vi "Vision.vi"() -> ()   [LabVIEW 2013]
uses:
  StateMachineStates 1.ctl
  <vilib>/DAQmx/read.llb/DAQmx Read (Counter DBL 1Chan 1Samp).vi
  <vilib>/DAQmx/create/channels.llb/DAQmx Create Channel (CI-Pulse Width).vi
  <vilib>/DAQmx/miscellaneous.llb/DAQmx Fill In Error Info.vi
panel:
  out "Triggered":bool
  in  "Use EEG trigger?":bool
  in  "Entrainment":bool=TRUE
  in  "Sound at \nstimulus end":bool
  in  "Manual \nvoltage (V)":dbl=2.6 format="%.2p"
  in  "Manual \nphoton #":i64=100
  out "L/R WP target":dbl
  out "List of axes":i32[](array[numeric])
  out "List of WP errors":bool[](array[boolean])
  out "WP error":bool
  out "appended array":dbl[][](array[numeric])
  out "Pump WP":dbl format="%.2f"
  in  "Trigger rate at \n52.6 degrees":dbl=2646.0 format="%.2p"
  in  "Target trial \nlength (ms)":dbl=500.0 format="%.2p"
  in  "Default pump \nWP angle":dbl=52.6
  in  "Pump WP":bool=TRUE
  out "Photon time (ms)":dbl format="%.2f"
  in  "Interval (ms)":u32
  out "Repetition":dbl
  in  "Repetitions":dbl=1.0
  out "WP time (ms)":u32
  out "VISA Handle out":refnum<visa-resource-name>="ASRL5::INSTR"
  out "Initializing":bool
  out "Trial mode":enum16{"Single Photons", "LED", "Mixed LED"}(ring)
  in  "Frequency of LED trials\nfor Mixed mode":dbl=30.0
  out "Bright trial\nrequested":bool
  out "Observer Ready":bool
  in  "Bright/mixed mode \nLED voltage (V)":dbl=2.6 min=-3.0 max=4.0 format="%.2f"
  in  "GPIB address":string="15"
  in  "Period (ms)":i64=20
  in  "Pulse \nlength (ms)":dbl=50.0
  out "L/R WP":dbl format="%.2f"
  in  "Manually \ninitialize":bool
  in  "COM for WPs":u8=3
  out "Blocked trial #":i32
  out "Photon #":i32
  out "LED Voltage":dbl
  in  "Blocking requirements":cluster{"Value":dbl, " Number":i32}[](array[cluster])
  in  "Manual":bool
  in  "Path":path=path "C:/Users/lab/Dropbox/Research/Data/Vision"
  out "Counts 2":u32
  out "Counts 1":u32
  in  "Delay for APDs (ms)":u32=25
  in  "Counter 2":tag="Dev1/ctr1"
  in  "Counter 1":tag="Dev1/ctr0"
  out "Trial #":i32
  in  "Mode":enum16{"Single Photons", "LED", "Mixed"}(ring)=enum."Mixed"
  in  "Audio":bool=TRUE
  in  "Self-paced":bool
  out "Stimulus":bool
  out "Location Set":bool
  out "Stimulus \nlocation":string
  out "Waiting":bool
  out "Observer Responded":bool
  out "Response \ntime (ms)":dbl
  out "Observer \nchoice":string
  out "Confidence":i32
  in  "stop":bool
  in  "Next Trial":bool
  in  "Create New File":bool
  out "Subject #":string
  # "Settings for Blocking\nand Mixed Mode"
  # "Instructions: Run VI. Enter blocking requirements, then press\nCreate New File. Initialize waveplates if necessary, and set\nhighlighted controls to desired values. Press Next Trial to begin."
  # "Researcher Interface"
  # "Trial Options"
  # "Counter Options"
  # "Trial Information"
  # "(1)"
  # "(3)"
  # "LED Options"
  # "Pump Settings"
  # "Troubleshooting"
  # "Waveplates"
  # "(2)"
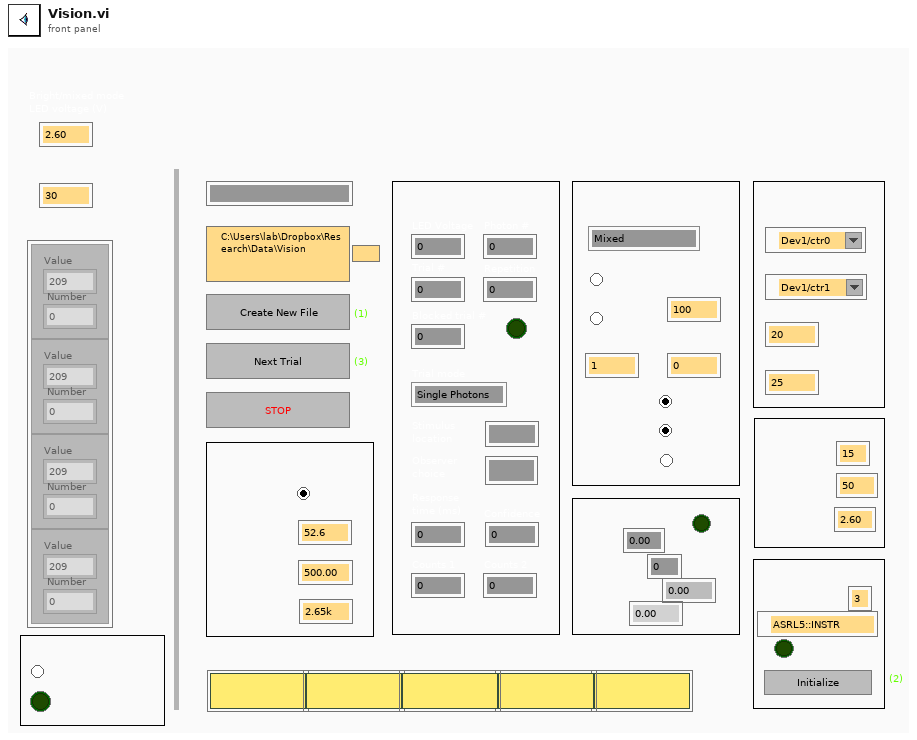
[diagram p1: front panel]
types:
  T1 = typedef "StateMachineStates 1.ctl" = enum16{"WaitResearcher", "Setup", "SetWP", "WaveplateError", "WaitObserverReady", "EEG", "Photons", "LED", "WaitObserverResponse", "CleanUp", "Stop"}
  T2 = enum16{"0", "1", "2", "3", "4", "5", "6", "7", "8", "9", "A", "B", "C", "D", "E", "F", "G", "H", "I", "J", "K", "L", "M", "N", "O", "P", "Q", "R", "S", "T", "U", "V", "W", "X", "Y", "Z", "F1", "F2", "F3", "F4", "F5", "F6", "F7", "F8", "F9", "F10", "F11", "F12", "F13", "F14", "F15", "ADD", "BACK", "BACKSLASH", "CAPITAL", "COMMA", "DECIMAL", "DELETE", "DIVIDE", "DOWN", "END", "EQUALS", "ESCAPE", "GRAVE (`)", "HOME", "INSERT", "LBRACKET", "LCONTROL", "LEFT", "L ALT", "LSHIFT", "LWIN", "MINUS", "MULTIPLY", "NEXT", "NUMLOCK", "NUMPAD_0", "NUMPAD_1", "NUMPAD_2", "NUMPAD_3", "NUMPAD_4", "NUMPAD_5", "NUMPAD_6", "NUMPAD_7", "NUMPAD_8", "NUMPAD_9", "PAUSE", "PERIOD", "PRIOR (PG UP)", "RBRACKET", "RCONTROL", "RETURN", "RIGHT", "R ALT", "RSHIFT", "RWIN", "SCROLL", "SEMICOLON", "SLASH", "SPACE", "SUBTRACT", "TAB", "UP", "ENTER (num pad)", "' (quote)"}
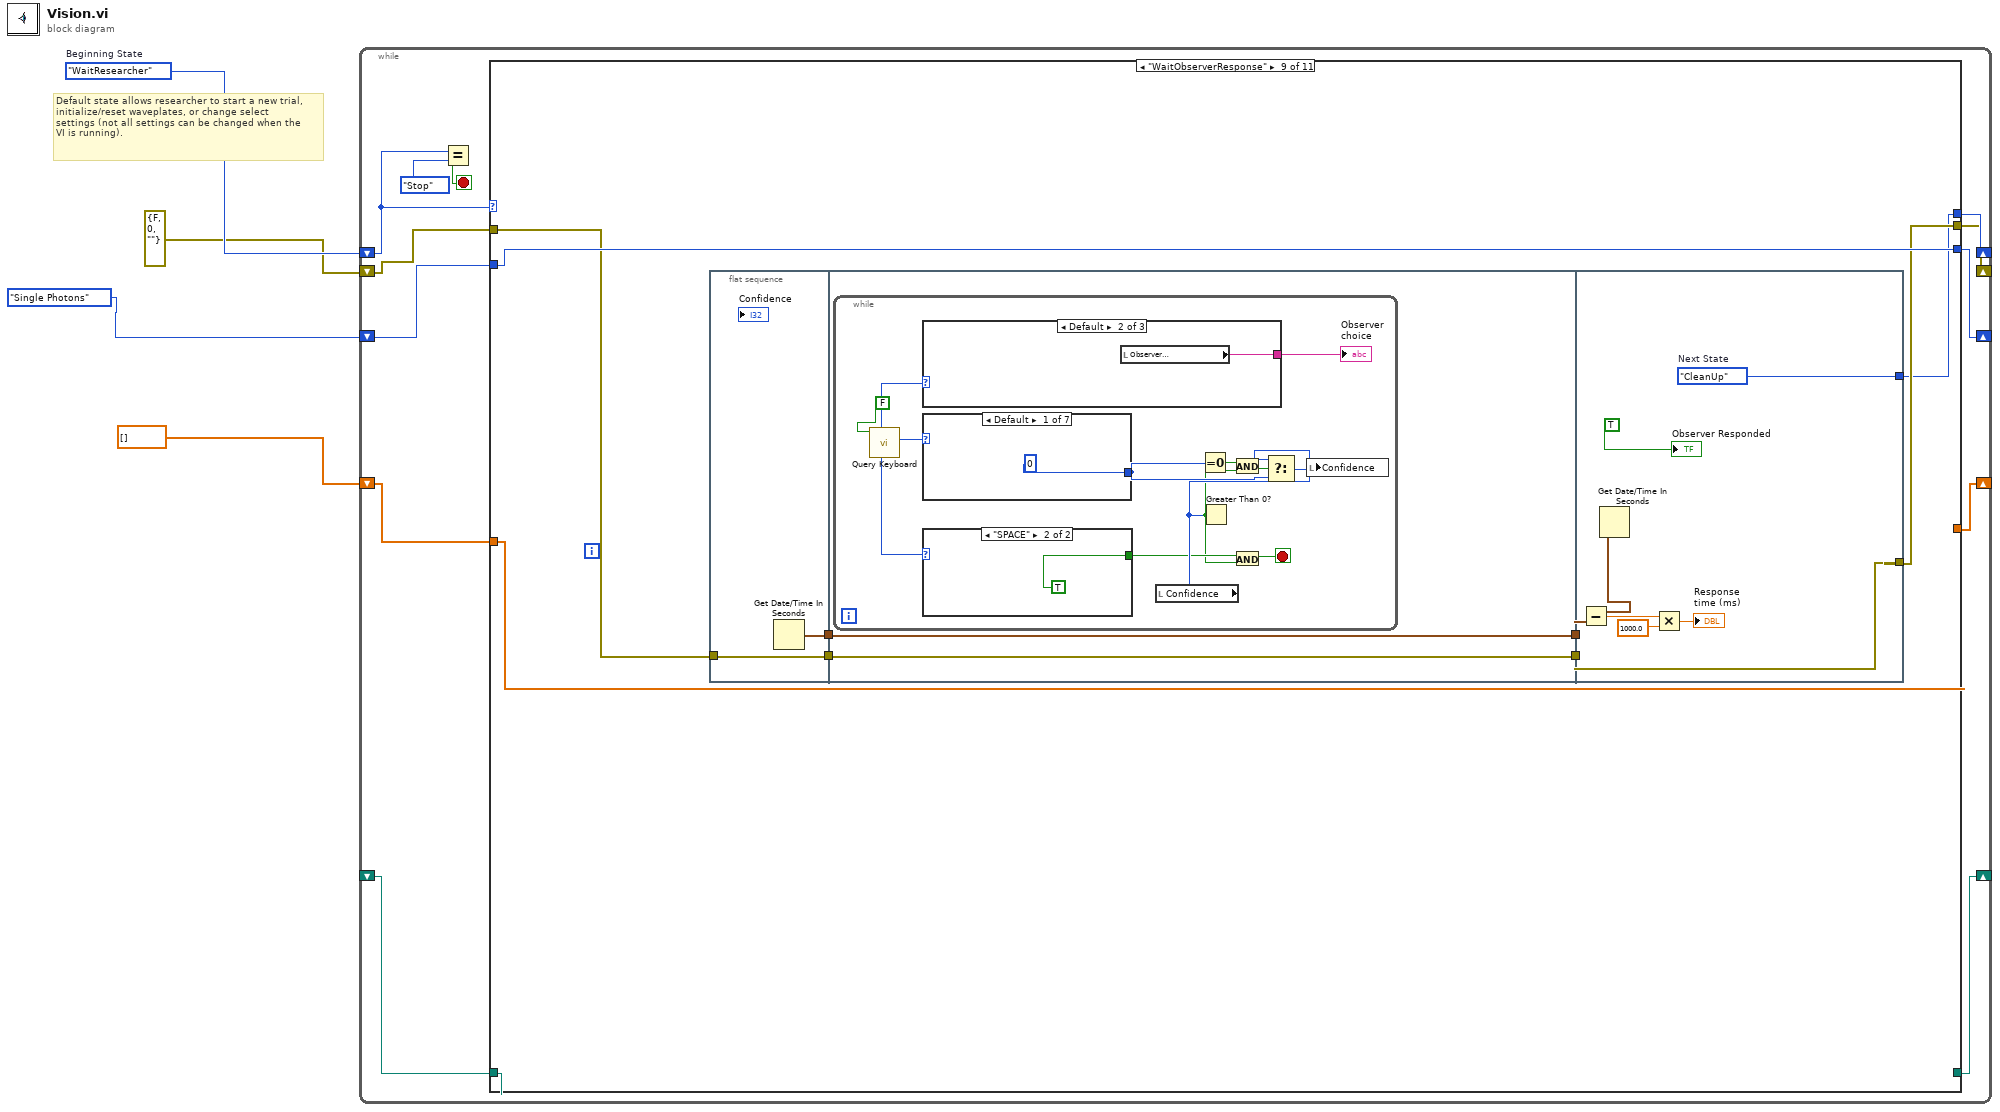
[diagram p0: block diagram]
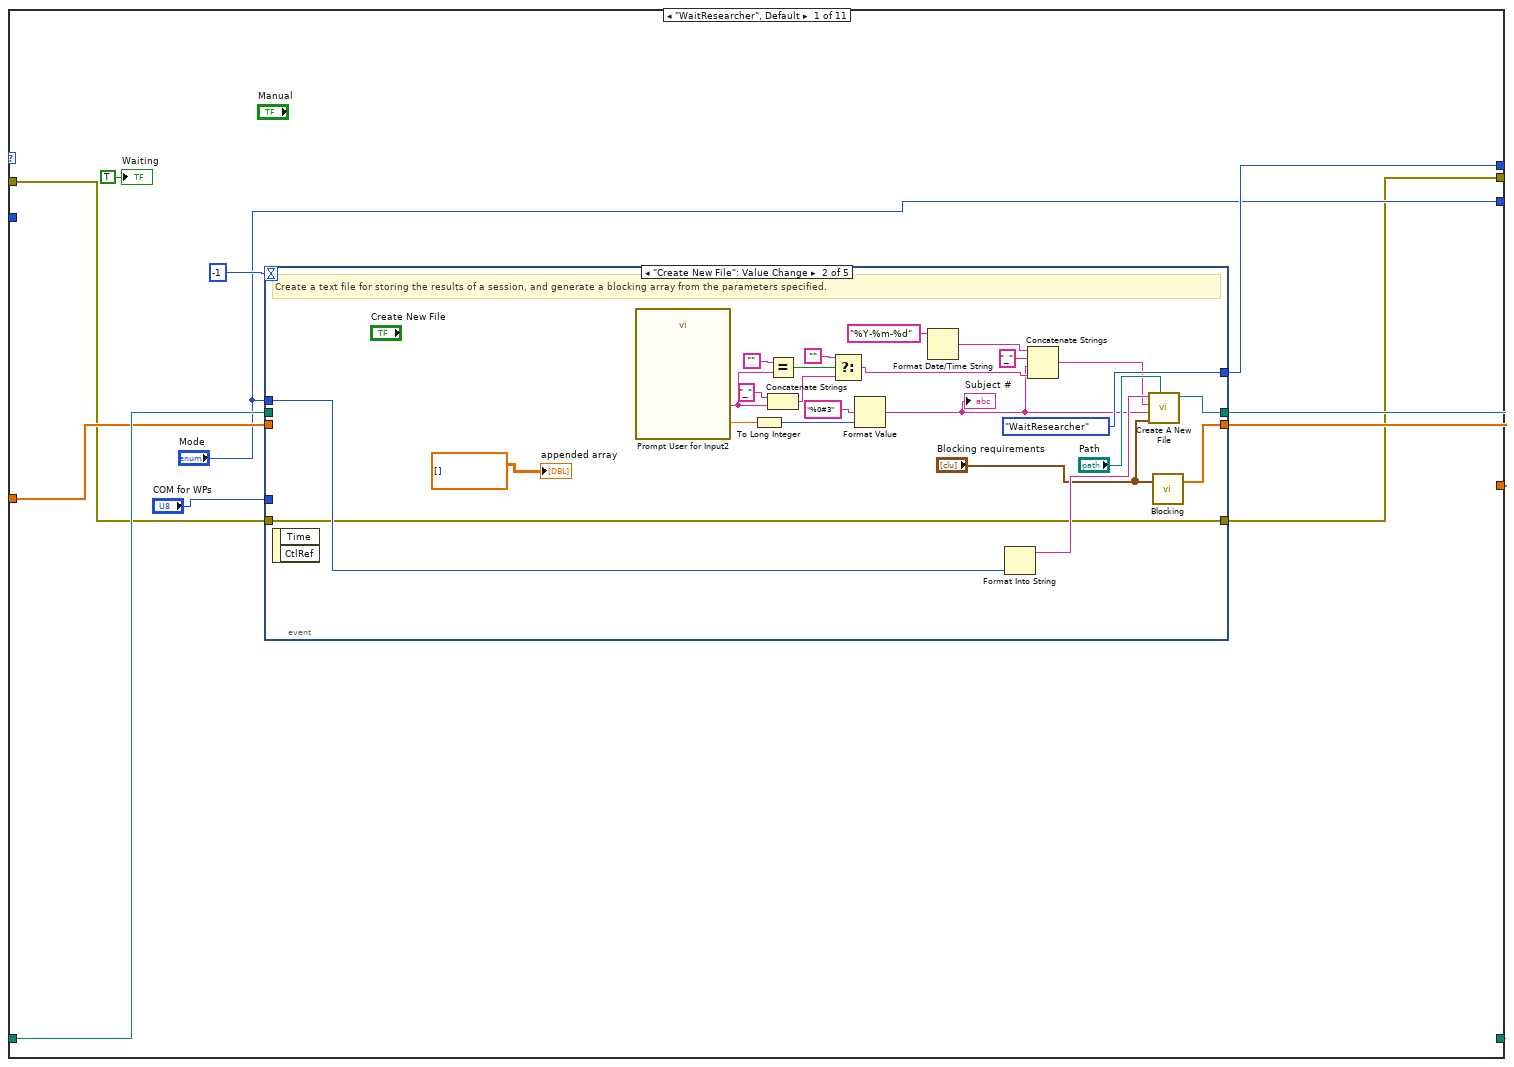
[diagram p2: hidden frame]
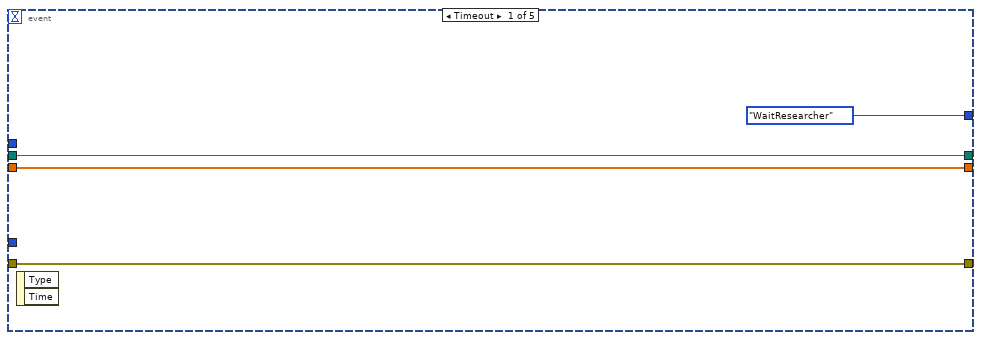
[diagram p3: hidden frame]
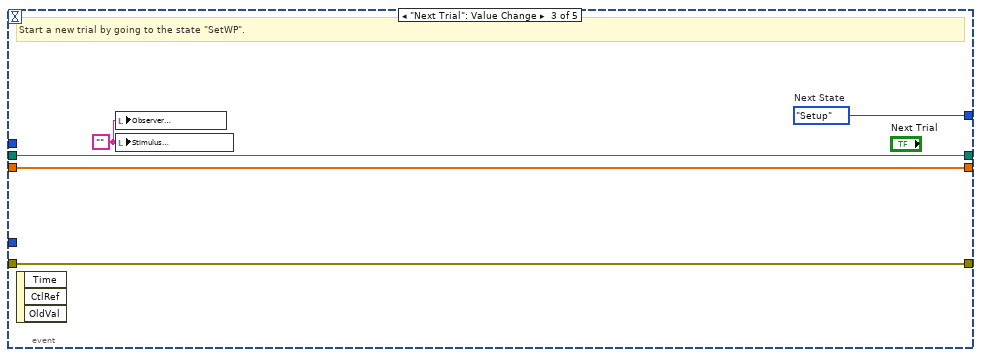
[diagram p4: hidden frame]
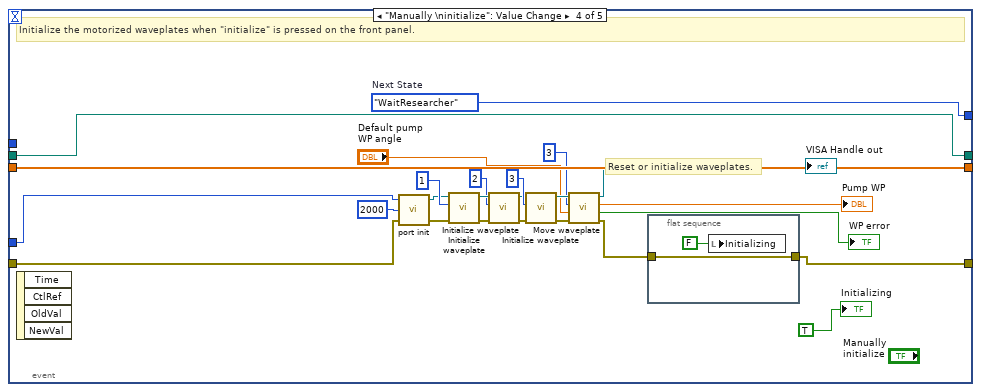
[diagram p5: hidden frame]
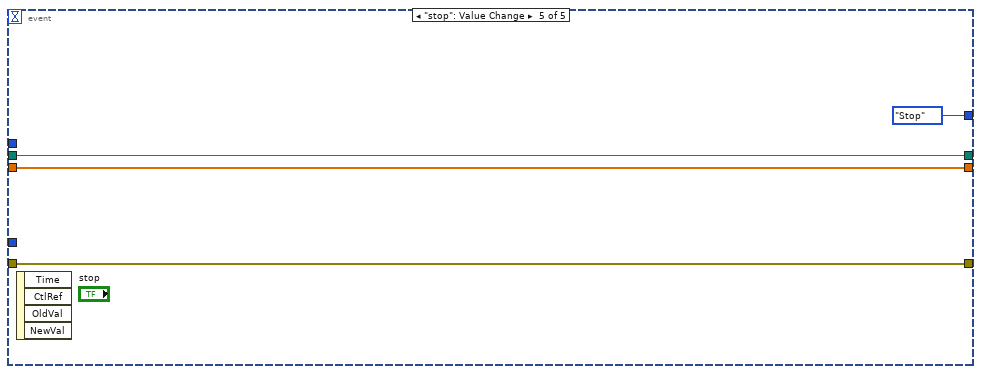
[diagram p6: hidden frame]
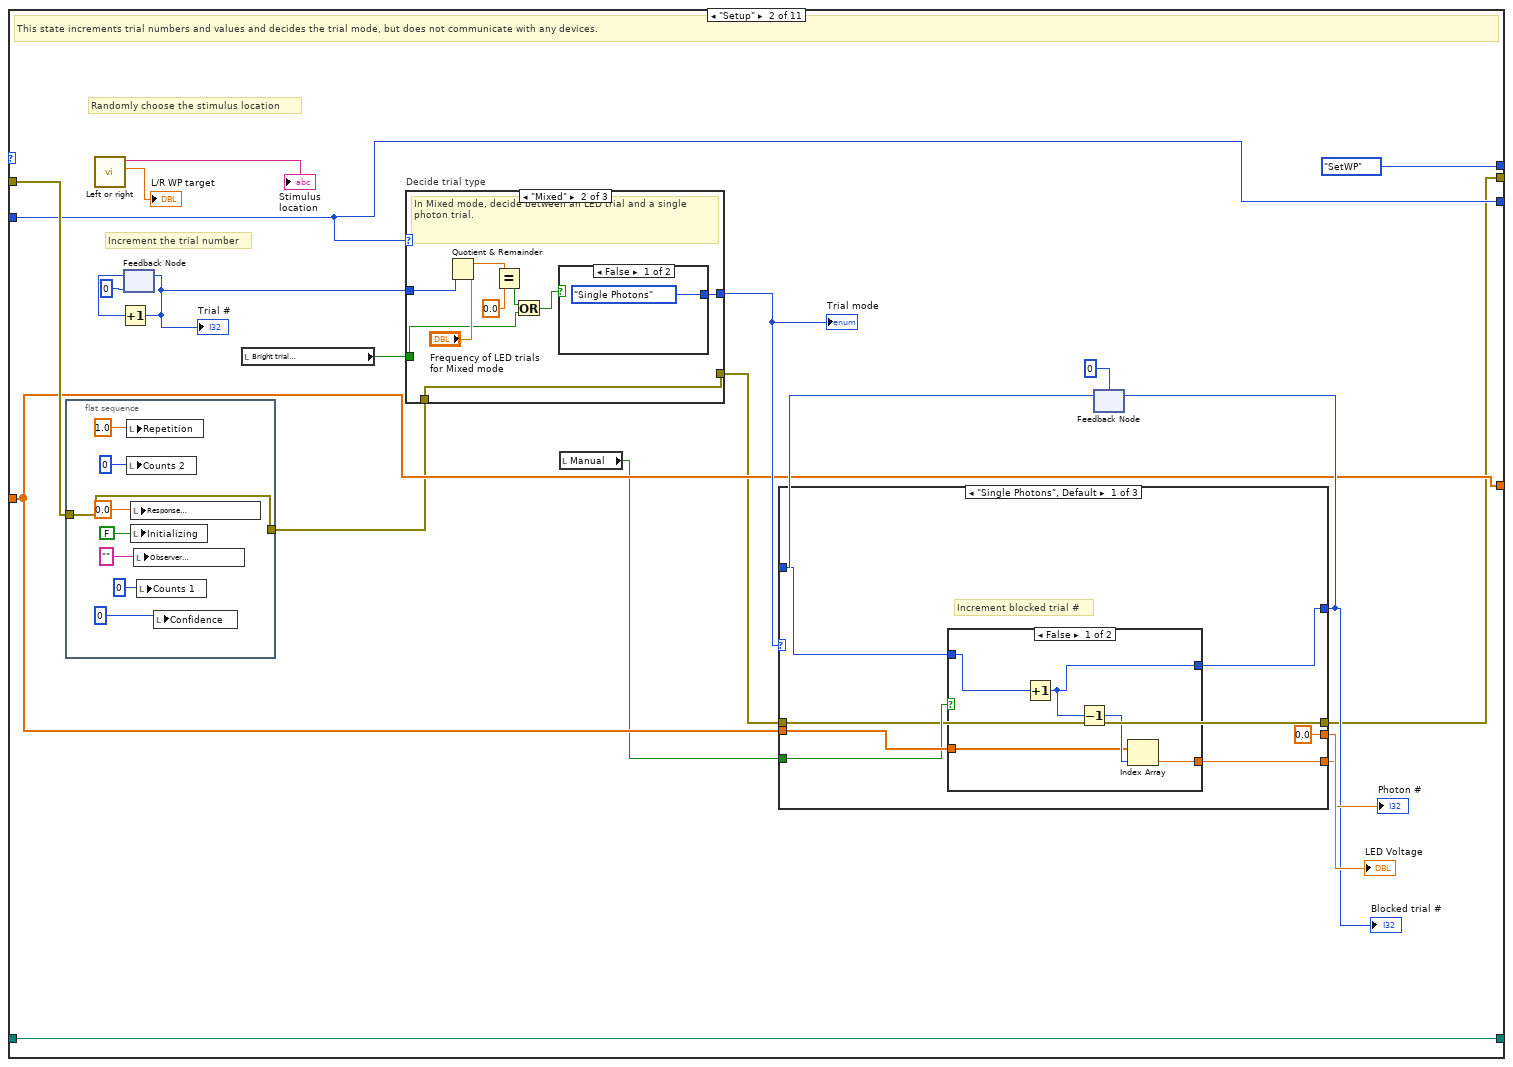
[diagram p7: hidden frame]
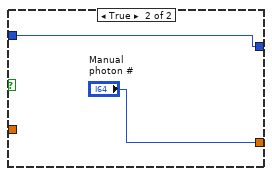
[diagram p8: hidden frame]
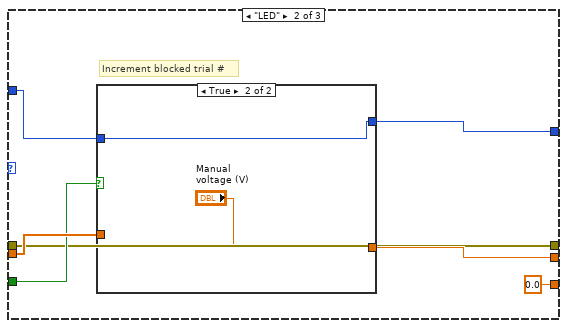
[diagram p9: hidden frame]
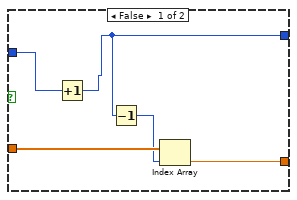
[diagram p10: hidden frame]
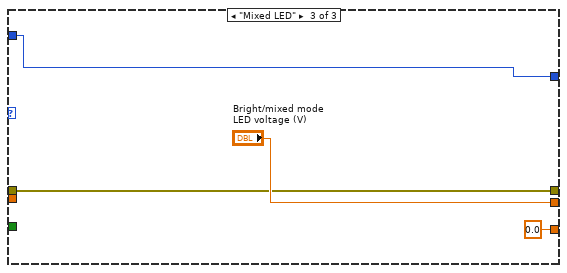
[diagram p11: hidden frame]
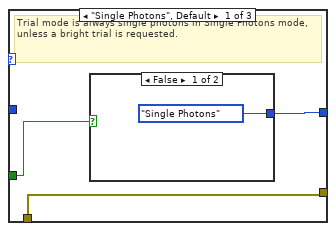
[diagram p12: hidden frame]
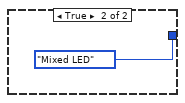
[diagram p13: hidden frame]
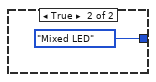
[diagram p14: hidden frame]
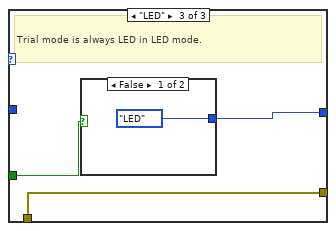
[diagram p15: hidden frame]
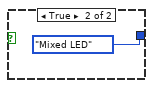
[diagram p16: hidden frame]
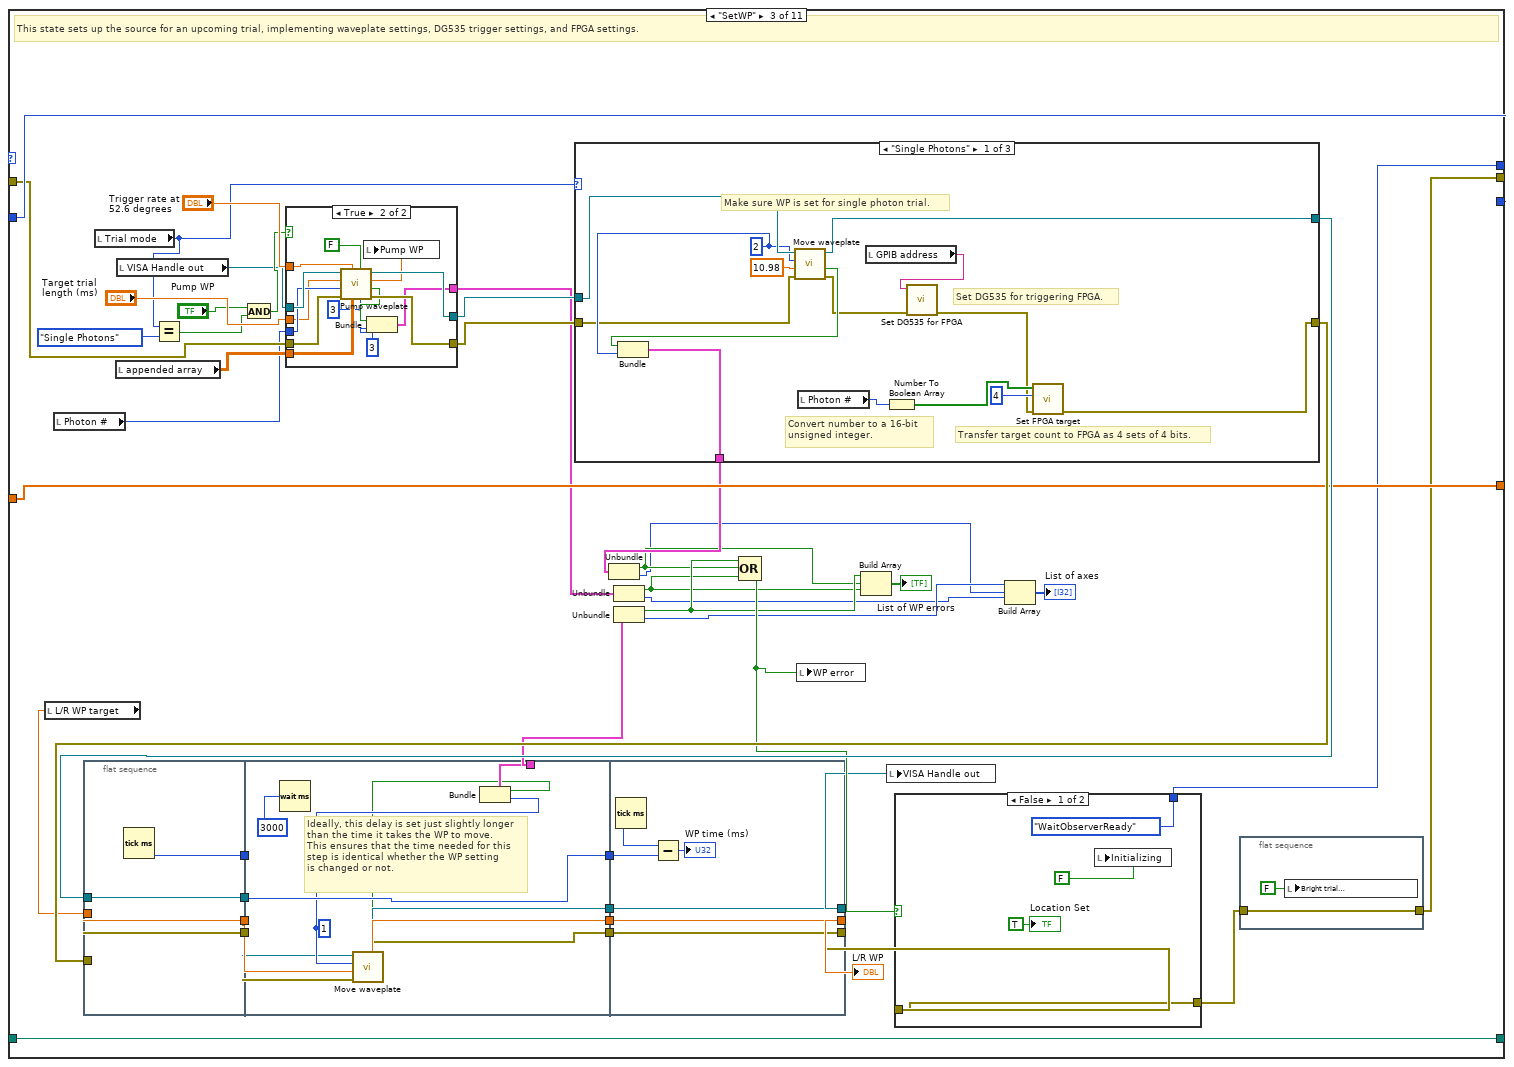
[diagram p17: hidden frame]
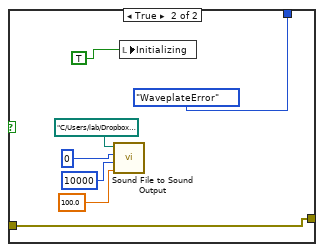
[diagram p18: hidden frame]
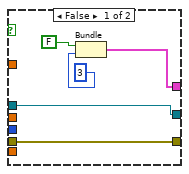
[diagram p19: hidden frame]
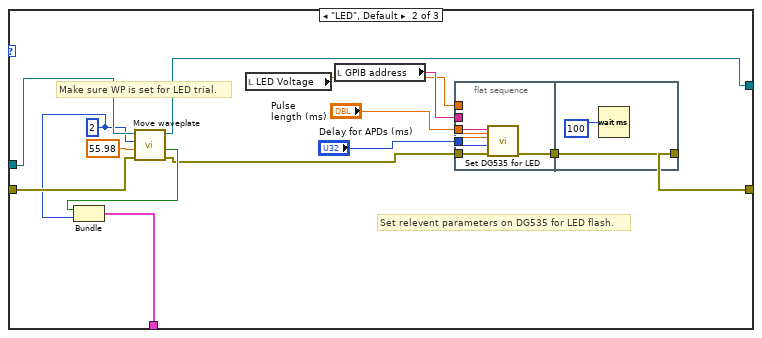
[diagram p20: hidden frame]
diagram:
  w4 = StateMachineStates_1."WaitResearcher"  # Beginning State
  # "Default state allows researcher to start a new trial,\ninitialize/reset waveplates, or change select\nsettings (not all settings can be changed when the\nVI is running)."
  n1 = while {
    shift-right: [w13] -> _
    shift-left: w4 -> [w14]
    shift-right: [w6] -> _
    shift-left: errorcluster {"status"=FALSE, "code"=0, "source"=""} ("error out") -> [w12]
    shift-right: [w11] -> _
    shift-left: enum16{"Single Photons", "LED", "Mixed"}."Single Photons" ("Mode") -> [w10]
    shift-right: [w9] -> _
    shift-left: _ -> [w5]
    shift-right: [w8] -> _
    shift-left: dbl[] [] ("Blocking array") -> [w7]
    stop <- w16 stop-if-true
    n2 = Equal?(x=w14, y=StateMachineStates_1."Stop" ("States")) -> (x = y?=w16:bool)
    n3 = case shown="\"WaitObserverResponse\"" w14 {
      selector: w14 -> [_ _ _ _ w387 _ _ _ _ _ _]
      tunnel: [w27 StateMachineStates_1."SetWP" ("Next State") w196 w336 w388 w424 StateMachineStates_1."WaitObserverResponse" ("Next State") w472 w486 w546 w584] -> w13
      tunnel: [w18 w93 w176 w333 w380 w426 w446 w468 w487 w537 w588] -> w6
      tunnel: w12 -> [w19 w111 w204 w337 w381 w426 w435 w451 w488 w536 w587]
      tunnel: ["Mode" w99 w216 w340 w385 w427 w442 w471 w493 w544 w591] -> w11
      tunnel: w10 -> [_ w99 w216 w340 w384 w427 w442 w471 w493 w544 w591]
      tunnel: [w24 w92 w217 w338 w383 w428 w439 w470 w492 w543 w590] -> w9
      tunnel: w5 -> [w23 w92 w217 w338 w383 w428 w439 w470 w492 w543 w590]
      tunnel: [w22 w98 w207 w339 w382 w429 w438 w469 w491 w541 w589] -> w8
      tunnel: w7 -> [w21 w98 w207 w339 w382 w429 w438 w469 w491 w541 w589]
      frame "WaitResearcher", Default {
        n4 = event shown="[1] \"Create New File\": Value Change" {
          selector: _ -> [_ _ _ _ _]
          dyn-events: _ -> [_ _ _ _ _]
          timeout: -1 -> [_ _ _ _ _]
          tunnel: [StateMachineStates_1."WaitResearcher" ("Next State") StateMachineStates_1."WaitResearcher" ("Next State") w56 w85 StateMachineStates_1."Stop" ("Next State")] -> w27
          tunnel: "Mode" -> [_ w51 _ _ _]
          tunnel: [w31 w45 w59 w84 w90] -> w24
          tunnel: w23 -> [w31 _ w59 w84 w90]
          tunnel: [w30 w49 w58 w82 w89] -> w22
          tunnel: w21 -> [w30 _ w58 w82 w89]
          tunnel: w19 -> [w29 w44 w57 w77 w88]
          tunnel: [w29 w44 w57 w81 w88] -> w18
          tunnel: "COM for WPs" -> [_ _ _ w78 _]
          event Timeout {
            n5 = event-data() -> ()  [unwired: 1 in, 2 out]
          }
          event "Create New File": Value Change {
            # "Create a text file for storing the results of a session, and generate a blocking array from the parameters specified."
            n6 = event-data() -> ()  [unwired: 1 in, 2 out]
            n7 = call "Prompt User for Input2"() -> ("Subject #"=w54:dbl, "Filename"=w39:string)  [unwired: 16 in, 2 out]
            n8 = To Long Integer(number=w54) -> (32bit integer=w35:i32)
            n9 = Equal?(x="", y=w39) -> (x = y?=w52:bool)
            n10 = Concatenate Strings("_" ("string"), w39) -> (w42:string)
            n11 = Select(t="", s=w52, f=w42) -> (s? t:f=w37:string)
            n12 = Format Value(format string="%0#3", value (0)=w35) -> (output string=w34:string)  [unwired: 1 in]
            "Subject #" <- w34
            n13 = Format Date/Time String(time format string (%c)="%Y-%m-%d") -> (date/time string=w40:string)  [unwired: 2 in]
            n14 = Format Into String(w51) -> (resulting string=w50:string)  [unwired: 3 in, 1 out]
            n15 = Concatenate Strings(w40, "_" ("string"), w34, w37) -> (w46:string)
            n16 = call "Create A New File.vi"("Path in"="Path", "Blocking requirements"="Blocking requirements", "Subject #"=w34, "Filename"=w46, "Mode"=w50) -> ("Path out"=w45:path)  [unwired: 6 in]
            n17 = call "Blocking.vi"("Blocking requirements"="Blocking requirements") -> ("Blocking array"=w49:dbl[])  [unwired: 2 in]
            "appended array" <- dbl[][] []
          }
          event "Next Trial": Value Change {
            w56 = StateMachineStates_1."Setup"  # Next State
            w60 = ""
            # "Start a new trial by going to the state \"SetWP\"."
            n18 = event-data() -> ()  [unwired: 1 in, 3 out]
            n19 = local write "Observer \nchoice"(w60) -> ()
            n20 = local write "Stimulus \nlocation"(w60) -> ()
          }
          event "Manually \ninitialize": Value Change {
            w85 = StateMachineStates_1."WaitResearcher"  # Next State
            # "Reset or initialize waveplates."
            # "Initialize the motorized waveplates when \"initialize\" is pressed on the front panel."
            n21 = event-data() -> ()  [unwired: 1 in, 4 out]
            n22 = call "port init.vi"("error in"=w77, "Timeout (ms)"=u32 2000 ("Timeout (300 ms)"), "SerialPort"=w78) -> ("error out"=w76:errorcluster, "Visa Handle"=w75:refnum<visa-resource-name>)  [unwired: 1 in]
            n23 = call "Initialize waveplate.vi"("error in (no error)"=w76, "Axis in"=1, "VISA Handle in"=w75) -> ("error out"=w72:errorcluster, "VISA Refnum out"=w74:refnum<visa-resource-name>)  [unwired: 6 in, 1 out]
            n24 = call "Initialize waveplate.vi"("error in (no error)"=w72, "Axis in"=2, "VISA Handle in"=w74) -> ("error out"=w69:errorcluster, "VISA Refnum out"=w70:refnum<visa-resource-name>)  [unwired: 6 in, 1 out]
            n25 = call "Initialize waveplate.vi"("error in (no error)"=w69, "Axis in"=3, "VISA Handle in"=w70) -> ("error out"=w65:errorcluster, "VISA Refnum out"=w68:refnum<visa-resource-name>)  [unwired: 6 in, 1 out]
            n26 = call "Move waveplate.vi"("error in (no error)"=w65, "Angle"="Default pump \nWP angle", "Axis in"=3, "VISA Refnum in"=w68) -> ("error out"=w64:errorcluster, "WP Error"=→"WP error":bool, "Current position (units)"=→"Pump WP":dbl, "VISA Refnum out"=→"VISA Handle out":refnum<visa-resource-name>)  [unwired: 4 in]
            n27 = flat-sequence {
              tunnel: w64 -> [w87]
              tunnel: [w87] -> w81
              frame #0 {
                n28 = local write "Initializing"(FALSE ("Initializing waveplates")) -> ()
              }
            }
            "Initializing" <- TRUE ("Initializing waveplates")
          }
          event "stop": Value Change {
            n29 = event-data() -> ()  [unwired: 1 in, 4 out]
          }
        }
        "Waiting" <- TRUE ("Waiting")
      }
      frame "Setup" {
        # "Randomly choose the stimulus location"
        # "Increment the trial number"
        # "This state increments trial numbers and values and decides the trial mode, but does not communicate with any devices."
        n30 = flat-sequence {
          tunnel: w111 -> [w145]
          tunnel: [w145] -> w95
          frame #0 {
            n31 = local write "Repetition"(1.0 ("Repitition #")) -> ()
            n32 = local write "Counts 2"(u32 0 ("Counts 2")) -> ()
            n33 = local write "Response \ntime (ms)"(0.0 ("Response \ntime (ms)")) -> ()
            n34 = local write "Initializing"(FALSE ("Initializing waveplates")) -> ()
            n35 = local write "Observer \nchoice"("" ("Observer \nchoice")) -> ()
            n36 = local write "Counts 1"(u32 0 ("Counts 1")) -> ()
            n37 = local write "Confidence"(0 ("Confidence")) -> ()
          }
        }
        n38 = call "Left or right.vi"() -> ("New target position (units)"=→"L/R WP target":dbl, "String"=→"Stimulus \nlocation":string)  [unwired: 10 in]
        n39 = feedback #1(0 ("x+1")) -> (w110:i32)
        n40 = Increment(x=w110) -> (x+1=w108:i32)
        "Trial #" <- w108
        n41 = feedback-in #1(w108) -> ()
        n42 = local read "Bright trial\nrequested"() -> (w100:bool)
        n43 = case "Decide trial type" shown="\"Mixed\"" w99 {
          tunnel: [w155 w165 w171] -> w107
          tunnel: w108 -> [_ w166 _]
          tunnel: w100 -> [w154 w159 w170]
          tunnel: w95 -> [w153 w158 w169]
          tunnel: [w153 w158 w169] -> w94
          frame "Single Photons", Default {
            # "Trial mode is always single photons in Single Photons mode, unless a bright trial is requested."
            n44 = case shown="False" w154 {
              tunnel: [enum16{"Single Photons", "LED", "Mixed LED"}."Single Photons" ("Mode") enum16{"Single Photons", "LED", "Mixed LED"}."Mixed LED" ("Mode")] -> w155
              frame False {
              }
              frame True {
              }
            }
          }
          frame "Mixed" {
            # "In Mixed mode, decide between an LED trial and a single photon trial."
            n45 = Quotient & Remainder(x=w166, y="Frequency of LED trials\nfor Mixed mode") -> (x-y*floor(x/y)=w163:dbl)  [unwired: 1 out]
            n46 = Equal?(x=w163, y=0.0) -> (x = y?=w161:bool)
            n47 = Or(x=w161, y=w159) -> (x .or. y?=w160:bool)
            n48 = case shown="False" w160 {
              tunnel: [enum16{"Single Photons", "LED", "Mixed LED"}."Single Photons" ("Mode") enum16{"Single Photons", "LED", "Mixed LED"}."Mixed LED" ("Mode")] -> w165
              frame False {
              }
              frame True {
              }
            }
          }
          frame "LED" {
            # "Trial mode is always LED in LED mode."
            n49 = case shown="False" w170 {
              tunnel: [enum16{"Single Photons", "LED", "Mixed LED"}."LED" ("Mode") enum16{"Single Photons", "LED", "Mixed LED"}."Mixed LED" ("Mode")] -> w171
              frame False {
              }
              frame True {
              }
            }
          }
        }
        "Trial mode" <- w107
        n50 = local read "Manual"() -> (w97:bool)
        n51 = feedback #2(0 ("x+1")) -> (w103:i32)
        n52 = case shown="\"Single Photons\", Default" w107 {
          tunnel: [w116 w132 w142] -> w102
          tunnel: w98 -> [w119 w133 _]
          tunnel: [0.0 ("Value") w131 "Bright/mixed mode \nLED voltage (V)"] -> w106
          tunnel: [w118 0.0 ("Value") 0.0 ("Value")] -> w105
          tunnel: w103 -> [w115 w129 w142]
          tunnel: w97 -> [w114 w128 _]
          tunnel: w94 -> [w113 w127 w141]
          tunnel: [w113 w127 w141] -> w93
          frame "Single Photons", Default {
            # "Increment blocked trial #"
            n53 = case shown="False" w114 {
              tunnel: w119 -> [w123 _]
              tunnel: [w122 "Manual \nphoton #"] -> w118
              tunnel: [w121 w125] -> w116
              tunnel: w115 -> [w120 w125]
              frame False {
                n54 = Increment(x=w120) -> (x+1=w121:i32)
                n55 = Decrement(x=w121) -> (x-1=w124:i32)
                n56 = Index Array(array=w123, index=w124) -> (element=w122:dbl)
              }
              frame True {
              }
            }
          }
          frame "LED" {
            # "Increment blocked trial #"
            n57 = case shown="True" w128 {
              tunnel: w133 -> [w138 _]
              tunnel: [w137 w139] -> w132
              tunnel: [w135 "Manual \nvoltage (V)"] -> w131
              tunnel: w129 -> [w134 w139]
              frame False {
                n58 = Increment(x=w134) -> (x+1=w137:i32)
                n59 = Decrement(x=w137) -> (x-1=w136:i32)
                n60 = Index Array(array=w138, index=w136) -> (element=w135:dbl)
              }
              frame True {
              }
            }
          }
          frame "Mixed LED" {
          }
        }
        "Photon #" <- w105
        "Blocked trial #" <- w102
        "LED Voltage" <- w106
        n61 = feedback-in #2(w102) -> ()
      }
      frame "SetWP" {
        # "This state sets up the source for an upcoming trial, implementing waveplate settings, DG535 trigger settings, and FPGA settings."
        n62 = local read "L/R WP target"() -> (w180:dbl)
        n63 = local read "Photon #"() -> (w181:i32)
        n64 = flat-sequence {
          tunnel: w215 -> [w253]
          tunnel: w214 -> [w254]
          tunnel: [w254] -> w213
          tunnel: [w253] -> w212
          tunnel: [w252] -> w208
          tunnel: w180 -> [w251]
          tunnel: [w251] -> w179
          tunnel: w213 -> [w262]
          tunnel: w212 -> [w259]
          tunnel: [w256] -> w211
          tunnel: [w257] -> w210
          tunnel: [w264] -> w209
          tunnel: w208 -> [w264]
          tunnel: [w263] -> w191
          tunnel: [w258] -> w182
          tunnel: w179 -> [w261]
          tunnel: [w269] -> w174
          tunnel: [w270] -> w195
          tunnel: [w271] -> w218
          tunnel: w211 -> [w270]
          tunnel: w210 -> [w269]
          tunnel: w209 -> [w268]
          tunnel: w182 -> [w271]
          frame #0 {
            n65 = Tick Count (ms)() -> (millisecond timer value=w252:u32)
          }
          frame #1 {
            w260 = 1 ("Axis in")
            # "Ideally, this delay is set just slightly longer\nthan the time it takes the WP to move.\nThis ensures that the time needed for this\nstep is identical whether the WP setting\nis changed or not."
            n66 = Wait (ms)(milliseconds to wait=u32 3000) -> ()  [unwired: 1 out]
            n67 = call "Move waveplate.vi"("error in (no error)"=w262, "Angle"=w261, "Axis in"=w260, "VISA Refnum in"=w259) -> ("error out"=w256:errorcluster, "WP Error"=w255:bool, "Current position (units)"=w258:dbl, "VISA Refnum out"=w257:refnum<visa-resource-name>)  [unwired: 4 in]
            n68 = Bundle("WP Error"=w255, "Axis in"=w260) -> (w263:cluster{"WP Error":bool, "Axis in":i32})  [unwired: 1 in]
          }
          frame #2 {
            n69 = Tick Count (ms)() -> (millisecond timer value=w267:u32)
            n70 = Subtract(x=w267, y=w268) -> (x-y=→"WP time (ms)":u32)
          }
        }
        n71 = local read "Trial mode"() -> (w178:enum16{"Single Photons", "LED", "Mixed LED"})
        n72 = local read "appended array"() -> (w201:dbl[][])
        n73 = local read "VISA Handle out"() -> (w175:refnum<visa-resource-name>)
        n74 = Equal?(x=w178, y=enum16{"Single Photons", "LED", "Mixed LED"}."Single Photons") -> (x = y?=w198:bool)
        n75 = And(x="Pump WP", y=w198) -> (x .and. y?=w197:bool)
        n76 = case shown="True" w197 {
          tunnel: w175 -> [w236 w250]
          tunnel: [w236 w249] -> w206
          tunnel: w204 -> [w235 w248]
          tunnel: [w235 w247] -> w205
          tunnel: w181 -> [_ w246]
          tunnel: "Target trial \nlength (ms)" -> [_ w245]
          tunnel: "Trigger rate at \n52.6 degrees" -> [_ w244]
          tunnel: w201 -> [_ w242]
          tunnel: [w233 w238] -> w192
          frame False {
            n77 = Bundle(FALSE, 3) -> (w233:cluster{bool, i32})  [unwired: 1 in]
          }
          frame True {
            n78 = call "Pump waveplate.vi"("Axis in"=3, "Trigger rate warnings?"=FALSE, "appended array"=w242, "Trigger rate \nat 52.6 degrees"=w244, "error in (no error)"=w248, "Photon #"=w246, "Target trial \nlength (ms)"=w245, "VISA Refnum in"=w250) -> ("error out"=w247:errorcluster, "WP Error"=w240:bool, "Current position (units)"=w243:dbl, "VISA Refnum out"=w249:refnum<visa-resource-name>)
            n79 = local write "Pump WP"(w243) -> ()
            n80 = Bundle("WP Error"=w240, 3) -> (w238:cluster{"WP Error":bool, i32})  [unwired: 1 in]
          }
        }
        n81 = case shown="\"Single Photons\"" w178 {
          tunnel: w205 -> [w279 w292 w312]
          tunnel: [w272 w295 w317] -> w214
          tunnel: w206 -> [w283 w293 w315]
          tunnel: [w277 w287 w309] -> w215
          tunnel: [w284 w294 w316] -> w193
          frame "Single Photons" {
            w281 = 2 ("Axis in")
            # "Convert number to a 16-bit\nunsigned integer."
            # "Transfer target count to FPGA as 4 sets of 4 bits."
            # "Set DG535 for triggering FPGA."
            # "Make sure WP is set for single photon trial."
            n82 = call "Move waveplate.vi"("error in (no error)"=w279, "Angle"=10.98 ("New target position (units)"), "Axis in"=w281, "VISA Refnum in"=w283) -> ("error out"=w278:errorcluster, "WP Error"=w280:bool, "VISA Refnum out"=w277:refnum<visa-resource-name>)  [unwired: 4 in, 1 out]
            n83 = Bundle("WP Error"=w280, "Axis in"=w281) -> (w284:cluster{"WP Error":bool, "Axis in":i32})  [unwired: 1 in]
            n84 = local read "Photon #"() -> (w275:i32)
            n85 = local read "GPIB address"() -> (w285:string)
            n86 = Number To Boolean Array(number=w275) -> (Boolean array=w274:bool[])
            n87 = call "Set DG535 for FPGA.vi"("error in (no error)"=w278, "GPIB address"=w285) -> ("error out"=w273:errorcluster)  [unwired: 9 in]
            n88 = call "Set FPGA target.vi"("error in (no error)"=w273, "Number of bits"=4, "Boolean array"=w274) -> ("error out"=w272:errorcluster)  [unwired: 8 in]
          }
          frame "LED", Default {
            w290 = 2 ("Axis in")
            # "Make sure WP is set for LED trial."
            # "Set relevent parameters on DG535 for LED flash."
            n89 = call "Move waveplate.vi"("error in (no error)"=w292, "Angle"=55.98 ("New target position (units)"), "Axis in"=w290, "VISA Refnum in"=w293) -> ("error out"=w288:errorcluster, "WP Error"=w289:bool, "VISA Refnum out"=w287:refnum<visa-resource-name>)  [unwired: 4 in, 1 out]
            n90 = Bundle("WP Error"=w289, "Axis in"=w290) -> (w294:cluster{"WP Error":bool, "Axis in":i32})  [unwired: 1 in]
            n91 = local read "LED Voltage"() -> (w286:dbl)
            n92 = local read "GPIB address"() -> (w299:string)
            n93 = flat-sequence {
              tunnel: "Delay for APDs (ms)" -> [w305]
              tunnel: w299 -> [w304]
              tunnel: "Pulse \nlength (ms)" -> [w303]
              tunnel: w286 -> [w302]
              tunnel: w288 -> [w301]
              tunnel: [w300] -> w296
              tunnel: w296 -> [w306]
              tunnel: [w306] -> w295
              frame #0 {
                n94 = call "Set DG535 for LED.vi"("amplitude"=w302, "error in"=w301, "Delay (ms)"=w305, "Pulse length (ms)"=w303, "GPIB address"=w304) -> ("error out"=w300:errorcluster)  [unwired: 6 in]
              }
              frame #1 {
                n95 = Wait (ms)(milliseconds to wait=u32 100) -> ()  [unwired: 1 out]
              }
            }
          }
          frame "Mixed LED" {
            w314 = 2 ("Axis in")
            # "Make sure WP is set for LED trial."
            n96 = local read "Bright/mixed mode \nLED voltage (V)"() -> (w308:dbl)
            n97 = call "Move waveplate.vi"("error in (no error)"=w312, "Angle"=55.98 ("New target position (units)"), "Axis in"=w314, "VISA Refnum in"=w315) -> ("error out"=w311:errorcluster, "WP Error"=w310:bool, "VISA Refnum out"=w309:refnum<visa-resource-name>)  [unwired: 4 in, 1 out]
            n98 = Bundle("WP Error"=w310, "Axis in"=w314) -> (w316:cluster{"WP Error":bool, "Axis in":i32})  [unwired: 1 in]
            n99 = local read "Delay for APDs (ms)"() -> (w319:u32)
            n100 = local read "Pulse \nlength (ms)"() -> (w320:dbl)
            n101 = local read "GPIB address"() -> (w321:string)
            n102 = flat-sequence {
              tunnel: w319 -> [w326]
              tunnel: w321 -> [w325]
              tunnel: w320 -> [w324]
              tunnel: w308 -> [w323]
              tunnel: w311 -> [w322]
              tunnel: [w322] -> w318
              tunnel: w318 -> [w327]
              tunnel: [w327] -> w317
              frame #0 {
                n103 = call "Set DG535 for LED.vi"("amplitude"=w323, "Delay (ms)"=w326, "Pulse length (ms)"=w324, "GPIB address"=w325) -> ()  [unwired: 7 in, 1 out]
              }
              frame #1 {
                n104 = Wait (ms)(milliseconds to wait=u32 100) -> ()  [unwired: 1 out]
              }
            }
          }
        }
        n105 = Unbundle(w193) -> ("WP Error"=w189:bool, "Axis in"=w185:i32)
        n106 = Unbundle(w192) -> ("WP Error"=w188:bool, w184:i32)
        n107 = Unbundle(w191) -> ("WP Error"=w190:bool, "Axis in"=w186:i32)
        n108 = Compound Arithmetic op=OR(w190, w189, w188) -> (w194:bool)
        n109 = local write "WP error"(w194) -> ()
        n110 = Build Array(w190, w189, w188) -> (→"List of WP errors":bool[])
        n111 = local write "VISA Handle out"(w174) -> ()
        n112 = case shown="False" w194 {
          tunnel: [StateMachineStates_1."WaitObserverReady" ("Next State") StateMachineStates_1."WaveplateError" ("Next State")] -> w196
          tunnel: w195 -> [w221 w229]
          tunnel: [w221 w229] -> w177
          frame False {
            n113 = local write "Initializing"(FALSE ("WP Error")) -> ()
            "Location Set" <- TRUE ("Location Set")
          }
          frame True {
            n114 = call "Sound File to Sound Output.vi"("Volume"=100.0, "Number of Samples/Iteration"=10000, "Device ID"=u32 0, "File Path"=path "C:/Users/lab/Dropbox/Vision software/Source/Windows Critical Stop.wav") -> ()
            n115 = local write "Initializing"(TRUE ("WP Error")) -> ()
          }
        }
        n116 = Build Array(w186, w185, w184) -> (→"List of axes":i32[])
        n117 = flat-sequence {
          tunnel: w177 -> [w220]
          tunnel: [w220] -> w176
          frame #0 {
            n118 = local write "Bright trial\nrequested"(FALSE ("Bright trial\nrequested")) -> ()
          }
        }
        "L/R WP" <- w218
      }
      frame "WaveplateError" {
        # "Resets waveplates in case of error in SetWP state."
        n119 = local read "VISA Handle out"() -> (w329:refnum<visa-resource-name>)
        n120 = call <vilib>:"Clear Errors.vi"("error in (no error)"=w337) -> ("error out"=w334:errorcluster)  [unwired: 6 in]
        n121 = local read "List of WP errors"() -> (w335:bool[])
        n122 = for {
          tunnel: w335 -> [w351] mode=indexing
          tunnel: w334 -> [w347]
          tunnel: [w346] -> w333
          tunnel: [w344] -> w331 mode=indexing
          shift-right: [w345] -> w332
          shift-left: w329 -> [w343]
          i -> [w349]
          n123 = local read "List of axes"() -> (w350:i32[])
          n124 = Index Array(array=w350, index=w349) -> (element=w348:i32)
          n125 = case shown="True" w351 {
            tunnel: w348 -> [_ w367]
            tunnel: w347 -> [w354 w368]
            tunnel: [w354 w364] -> w346
            tunnel: w343 -> [w353 w363]
            tunnel: [w353 w361] -> w345
            tunnel: [FALSE ("WP Error") w356] -> w344
            frame False {
            }
            frame True {
              n126 = local read "Pump WP"() -> (w358:bool)
              n127 = Not(x=w358) -> (.not. x?=w357:bool)
              n128 = call "Initialize waveplate.vi"("error in (no error)"=w368, "Axis in"=w367, "VISA Handle in"=w363) -> ("error out"=w365:errorcluster, "WP Error"=w355:bool, "VISA Refnum out"=w362:refnum<visa-resource-name>)  [unwired: 6 in]
              n129 = Equal?(x=3, y=w367) -> (x = y?=w360:bool)
              n130 = And(x=w357, y=w360) -> (x .and. y?=w359:bool)
              n131 = case shown="True" w359 {
                tunnel: w365 -> [w371 w376]
                tunnel: [w371 w375] -> w364
                tunnel: w362 -> [w370 w374]
                tunnel: [w370 w373] -> w361
                tunnel: [w369 w372] -> w356
                tunnel: w355 -> [w369 _]
                frame False {
                }
                frame True {
                  n132 = local read "Default pump \nWP angle"() -> (w378:dbl)
                  n133 = call "Move waveplate.vi"("error in (no error)"=w376, "Angle"=w378, "Axis in"=3, "VISA Refnum in"=w374) -> ("error out"=w375:errorcluster, "WP Error"=w372:bool, "Current position (units)"=w379:dbl, "VISA Refnum out"=w373:refnum<visa-resource-name>)  [unwired: 4 in]
                  n134 = local write "Pump WP"(w379) -> ()
                }
              }
            }
          }
        }
        n135 = local write "VISA Handle out"(w332) -> ()
        n136 = Or Array Elements(Boolean array=w331) -> (logical OR=w330:bool)
        n137 = case shown="True" w330 {
          tunnel: [StateMachineStates_1."SetWP" ("Next State") StateMachineStates_1."WaveplateError" ("Next State")] -> w336
          frame False {
          }
          frame True {
          }
        }
      }
      frame "WaitObserverReady" {
        # "Wait for the observer to trigger the beginning of a trial by pressing the spacebar, then go to a stimulus-producing state determined by \"mode\" on the front panel."
        n138 = flat-sequence {
          tunnel: [w390] -> w386
          tunnel: w381 -> [w390]
          tunnel: w387 -> [w401]
          tunnel: w386 -> [w399]
          tunnel: w384 -> [w394]
          tunnel: [w395] -> w380
          tunnel: [w402] -> w388
          tunnel: [w398] -> w385
          frame #0 {
            n139 = local read "Bright/mixed mode \nLED voltage (V)"() -> (w389:dbl)
            n140 = local read "LED Voltage"() -> (w391:dbl)
            n141 = call "Play sound start trial.vi"("LED Voltage"=w391, "Bright/mixed mode \nLED voltage (V)"=w389) -> ()  [unwired: 10 in]
          }
          frame #1 {
            n142 = local read "Trial mode"() -> (w393:enum16{"Single Photons", "LED", "Mixed LED"})
            n143 = call "Query Keyboard.vi"("error in (no error)"=w399, "Stop?"=FALSE) -> ("error out"=w396:errorcluster, "element"=w400:T2)  [unwired: 8 in]
            n144 = case shown="\"SPACE\"" w400 {
              tunnel: [StateMachineStates_1."WaitObserverReady" ("Next State") w412 StateMachineStates_1."WaitObserverReady" ("Next State")] -> w402
              tunnel: w401 -> [_ _ _]
              tunnel: [w405 w411 w422] -> w398
              tunnel: w394 -> [w405 w411 w422]
              tunnel: w396 -> [w404 w410 w419]
              tunnel: [w404 w410 w419] -> w395
              tunnel: w393 -> [_ w409 _]
              tunnel: [FALSE ("Observer Ready") TRUE ("Observer Ready") FALSE ("Observer Ready")] -> w392
              frame "1", Default {
              }
              frame "SPACE" {
                # "If the subject presses SPACE, move to the appropriate stimulus-producing mode (either Photons, Detectors, or LED)."
                n145 = case shown="False" "Use EEG trigger?" {
                  tunnel: [w414 w418] -> w412
                  tunnel: w409 -> [w413 _]
                  frame False {
                    n146 = case shown="\"Mixed LED\"" w413 {
                      tunnel: [w415 w416 w417] -> w414
                      frame "Single Photons", Default {
                        w415 = StateMachineStates_1."Photons"  # Next State
                      }
                      frame "LED" {
                        w416 = StateMachineStates_1."LED"  # Next State
                      }
                      frame "Mixed LED" {
                        w417 = StateMachineStates_1."LED"  # Next State
                      }
                    }
                  }
                  frame True {
                    w418 = StateMachineStates_1."Photons"  # Next State
                  }
                }
              }
              frame "NUMPAD_0" {
                # "If the subject presses 0, set the \"bright trial requested\" flag and keep waiting for a response"
                "Bright trial\nrequested" <- TRUE ("Bright trial\nrequested")
              }
            }
            "Observer Ready" <- w392
          }
        }
      }
      frame "EEG" {
        n147 = call "EEGstatus.vi"() -> ("Is minima found?"=w425:bool)  [unwired: 11 in]
        n148 = local write "Triggered"(w425) -> ()
        n149 = event shown="[1] \"Triggered\": Value Change" {
          selector: _ -> [_ _]
          dyn-events: _ -> [_ _]
          timeout: _ -> [_ _]
          tunnel: [_ w431] -> w424
          event Timeout {
            n150 = event-data() -> ()  [unwired: 1 in, 3 out]
          }
          event "Triggered": Value Change {
            n151 = event-data() -> ()  [unwired: 1 in, 6 out]
            n152 = local read "Trial mode"() -> (w430:enum16{"Single Photons", "LED", "Mixed LED"})
            n153 = case shown="\"Single Photons\", Default" w430 {
              tunnel: [w432 w433 w434] -> w431
              frame "Single Photons", Default {
                w432 = StateMachineStates_1."Photons"  # Next State
              }
              frame "LED" {
                w433 = StateMachineStates_1."LED"  # Next State
              }
              frame "Mixed LED" {
                w434 = StateMachineStates_1."LED"  # Next State
              }
            }
          }
        }
      }
      frame "LED" {
        # "Flash LED while reading out counts from two single-photon detectors."
        n154 = call "flashLED_DG535andcount.vi"("error in"=w435, "GPIB address"="GPIB address", "Period"="Period (ms)", "Counter 2"="Counter 2", "Counter 1"="Counter 1") -> ("Counts 2"=→"Counts 2":u32, "Counts 1"=→"Counts 1":u32, "error out"=w445:errorcluster)  [unwired: 4 in]
        n155 = flat-sequence {
          tunnel: w445 -> [w448]
          tunnel: [w448] -> w446
          frame #0 {
            "Stimulus" <- TRUE ("Stimulus")
          }
        }
      }
      frame "Photons" {
        w461 = 30.0  # timeout
        w458 = 10280 items=["Rising"=10280, "Falling"=10171] ("Starting Edge")
        # "This sets up the DAQ card to measure the duration of the trial (how long the FPGA is counting photons before it reaches the target number)."
        n156 = local read "Repetition"() -> (w465:dbl)
        n157 = call-poly <vilib>:"DAQmx Create Virtual Channel.vi"("maximum value"=5.0 ("Maximum Value (sec)"), "minimum value"=0.001 ("Minimum Value (sec)"), "counter"=tag "Dev1/ctr3" ("Physical Channel"), "error in"=w451, "starting edge"=w458) -> ("task out"=w457:refnum<k21>, "error out"=w452:errorcluster)  [unwired: 9 in]
        n158 = Greater Or Equal?(x=w465, y="Repetitions") -> (x >= y?=w467:bool)
        n159 = call "Count photons with FPGA.vi"("error in (no error)"=w452, "Entrainment"="Entrainment") -> ("error out"=w464:errorcluster)  [unwired: 9 in]
        n160 = case shown="True" w467 {
          tunnel: [StateMachineStates_1."Photons" ("States") StateMachineStates_1."WaitObserverResponse" ("States")] -> w472
          tunnel: w464 -> [w476 w480]
          tunnel: [w476 w480] -> w468
          tunnel: w465 -> [w475 _]
          frame False {
            n161 = Increment(x=w475) -> (x+1=→"Repetition":dbl)
            n162 = Wait (ms)(milliseconds to wait="Interval (ms)") -> ()  [unwired: 1 out]
          }
          frame True {
            n163 = local write "Stimulus"(TRUE ("Counts Taken")) -> ()
            n164 = case shown="True" "Sound at \nstimulus end" {
              frame False {
              }
              frame True {
                n165 = call "Sound File to Sound Output.vi"("Volume"=100.0, "Number of Samples/Iteration"=10000, "Device ID"=u32 0, "File Path"=path "C:/Users/Lab/Dropbox/Vision software/Speech Misrecognition.wav") -> ()
              }
            }
          }
        }
        n166 = call-poly <vilib>:"DAQmx Read.vi"("task/channels in"=w457, "timeout"=w461) -> ("task out"=w459:refnum<k21>, "data"=w463:dbl, "error out"=w460:errorcluster)  [unwired: 11 in]
        n167 = call <vilib>:"DAQmx Clear Task.vi"("task in"=w459, "error in"=w460) -> ()  [unwired: 13 in, 1 out]
        n168 = Multiply(x=w463, y=1000.0) -> (x*y=→"Photon time (ms)":dbl)
      }
      frame "WaitObserverResponse" {
        n169 = flat-sequence {
          tunnel: [w497] -> w495
          tunnel: w488 -> [w496]
          tunnel: [w496] -> w489
          tunnel: [w499] -> w494
          tunnel: w495 -> [w499]
          tunnel: [w498] -> w490
          tunnel: w489 -> [w498]
          tunnel: [w530] -> w486
          tunnel: w494 -> [w525]
          tunnel: [w523] -> w487
          tunnel: w490 -> [w523]
          frame #0 {
            n170 = Get Date/Time In Seconds() -> (seconds since 1Jan1904=w497:timestamp)
          }
          frame #1 {
            n171 = while {
              stop <- w503 stop-if-true
              n172 = call "Query Keyboard.vi"("Stop?"=FALSE) -> ("element"=w501:T2)  [unwired: 9 in, 1 out]
              n173 = case shown="Default" w501 {
                tunnel: ["Left" w512 "Right"] -> w502
                frame "D", "F", "S" {
                }
                frame Default {
                  n174 = local read "Observer \nchoice"() -> (w512:string)
                }
                frame "J".."L" {
                }
              }
              "Observer \nchoice" <- w502
              n175 = case shown="Default" w501 {
                tunnel: [0 1 2 3 3 2 1] -> w507
                frame Default {
                }
                frame "S" {
                }
                frame "D" {
                }
                frame "F" {
                }
                frame "J" {
                }
                frame "K" {
                }
                frame "L" {
                }
              }
              n176 = case shown="\"SPACE\"" w501 {
                tunnel: [FALSE TRUE] -> w505
                frame "0", Default {
                }
                frame "SPACE" {
                }
              }
              n177 = local read "Confidence"() -> (w506:i32)
              n178 = Equal To 0?(x=w507) -> (x = 0?=w509:bool)
              n179 = Greater Than 0?(x=w506) -> (x > 0?=w504:bool)
              n180 = And(x=w509, y=w504) -> (x .and. y?=w508:bool)
              n181 = And(x=w505, y=w504) -> (x .and. y?=w503:bool)
              n182 = Select(t=w506, s=w508, f=w507) -> (s? t:f=w510:i32)
              n183 = local write "Confidence"(w510) -> ()
            }
          }
          frame #2 {
            w530 = StateMachineStates_1."CleanUp"  # Next State
            n184 = Get Date/Time In Seconds() -> (seconds since 1Jan1904=w528:timestamp)
            n185 = Subtract(x=w528, y=w525) -> (x-y=w527:dbl)
            n186 = Multiply(x=w527, y=1000.0) -> (x*y=→"Response \ntime (ms)":dbl)
            "Observer Responded" <- TRUE ("Boolean 3")
          }
        }
      }
      frame "CleanUp" {
        n187 = local read "Manual"() -> (w532:bool)
        n188 = local read "Stimulus \nlocation"() -> (w534:string)
        n189 = local read "Observer \nchoice"() -> (w531:string)
        n190 = local read "Blocked trial #"() -> (w533:i32)
        n191 = flat-sequence {
          tunnel: w534 -> [w562]
          tunnel: w531 -> [w561]
          tunnel: w543 -> [w560]
          tunnel: w536 -> [w558]
          tunnel: [w558] -> w535
          frame #0 {
            # "Write data from trial to file."
            n192 = local read "Subject #"() -> (w547:string)
            n193 = Equal?(x=w562, y=w561) -> (x = y?=w564:bool)
            n194 = local read "Trial #"() -> (w551:i32)
            n195 = local read "Counts 2"() -> (w549:u32)
            n196 = local read "Counts 1"() -> (w548:u32)
            n197 = local read "Confidence"() -> (w550:i32)
            n198 = local read "Photon #"() -> (w557:i32)
            n199 = local read "Response \ntime (ms)"() -> (w563:dbl)
            n200 = local read "Photon time (ms)"() -> (w556:dbl)
            n201 = local read "LED Voltage"() -> (w559:dbl)
            n202 = local read "Pump WP"() -> (w552:dbl)
            n203 = call "Prepare data and write to file.vi"("Photon time (ms)"=w556, "String"=w562, "Confidence"=w550, "Photon #"=w557, "Pump WP"=w552, "Observer choice"=w561, "LED Voltage"=w559, "Response \ntime (ms)"=w563, "Path in"=w560, "Boolean"=w564, 10:w551, "Counts in"=w548, "Subject #"=w547, "Counts 1"=w549) -> ()  [unwired: 6 in]
            n204 = feedback #3() -> (w555:dbl[][])  [unwired: 1 in]
            n205 = Build Array(w557, w556, w552) -> (w554:dbl[])
            n206 = Build Array (concatenate)(w554, w555) -> (w553:dbl[][])
            n207 = local write "appended array"(w553) -> ()
            n208 = feedback-in #3(w553) -> ()
          }
        }
        n209 = Array Size(array=w541) -> (size(s)=w540:i32)
        n210 = call "Play sound right wrong.vi"("Audio"="Audio", "String"=w534, "Observer choice"=w531) -> ()  [unwired: 9 in]
        n211 = Equal?(x=w540, y=w533) -> (x = y?=w539:bool)
        n212 = Not(x=w532) -> (.not. x?=w542:bool)
        n213 = And(x=w542, y=w539) -> (x .and. y?=w538:bool)
        n214 = case shown="False" w538 {
          tunnel: [w569 w578] -> w546
          tunnel: w532 -> [_ _]
          frame False {
            # "Display a message and\nswitch to manual mode\nif end of blocked trials\nis reached."
            n215 = case shown="True" "Self-paced" {
              tunnel: [w571 w575] -> w569
              frame False {
                n216 = call "Display Message to User"() -> ("OK"=w570:bool)  [unwired: 10 in, 1 out]
                n217 = case shown="True" w570 {
                  tunnel: [w572 w574] -> w571
                  frame False {
                    w572 = StateMachineStates_1."CleanUp"  # Next State
                  }
                  frame True {
                    w574 = StateMachineStates_1."WaitResearcher"  # Next State
                    n218 = local write "Observer Responded"(FALSE ("Observer Responded")) -> ()
                  }
                }
              }
              frame True {
                w575 = StateMachineStates_1."Setup"  # Next State
                # "Skip \"WaitingResearcher\" mode if trials are self-paced."
                n219 = local write "Observer Responded"(FALSE ("Observer Responded")) -> ()
              }
            }
          }
          frame True {
            n220 = local write "Self-paced"(FALSE ("Self-paced")) -> ()
            n221 = call "Display Message to User2"() -> ("OK"=w579:bool)  [unwired: 10 in, 1 out]
            n222 = case shown="False" w579 {
              tunnel: [w581 w583] -> w578
              frame False {
                w581 = StateMachineStates_1."CleanUp"  # Next State
              }
              frame True {
                w583 = StateMachineStates_1."WaitResearcher"  # Next State
                n223 = local write "Observer Responded"(FALSE ("Observer Responded")) -> ()
              }
            }
            n224 = local write "Manual"(TRUE ("Manual")) -> ()
          }
        }
        n225 = flat-sequence {
          tunnel: [w565] -> w537
          tunnel: w535 -> [w565]
          frame #0 {
            w567 = FALSE ("LC")
            # "Reset indicators"
            n226 = local write "LED Voltage"(0.0 ("LED Voltage")) -> ()
            n227 = local write "Location Set"(w567) -> ()
            n228 = local write "Waiting"(w567) -> ()
            n229 = local write "Stimulus"(w567) -> ()
            n230 = local write "Observer Ready"(w567) -> ()
          }
        }
      }
      frame "Stop" {
        n231 = flat-sequence {
          tunnel: w587 -> [w593]
          tunnel: [w594] -> w586
          tunnel: w586 -> [w596]
          tunnel: [w596] -> w585
          tunnel: [w598] -> w588
          tunnel: w585 -> [w598]
          tunnel: [StateMachineStates_1."Stop" ("Next State")] -> w584
          frame #0 {
            # "Close waveplate session."
            n232 = local read "VISA Handle out"() -> (w592:refnum<visa-resource-name>)
            n233 = call "close.vi"("error in"=w593, "VISA Handle in"=w592) -> ("error out"=w594:errorcluster)  [unwired: 3 in]
          }
          frame #1 {
            w595 = FALSE ("LC")
            # "Reset indicator lights."
            n234 = local write "Stimulus"(w595) -> ()
            n235 = local write "Location Set"(w595) -> ()
            n236 = local write "Observer Responded"(w595) -> ()
            n237 = local write "Waiting"(w595) -> ()
            n238 = local write "Observer Ready"(w595) -> ()
          }
          frame #2 {
          }
        }
      }
    }
  }
